vi "Value with no SI Prefix To Value with SI prefix.vi"(7 "Output Prefix":T1, 8 "error in":errorcluster, 10 "Unit In":T2, 11 "Scaled Value":dbl format="%#.6f") -> (0 "error out":errorcluster, 2 "Unit (with prefix)":T2, 3 "Value":dbl format="%#.6f")   [LabVIEW 2013, in "Mercury iXX.lvlib"]
doc: "This VI converts a numeric input in base units into a numeric with a user-selectable SI prefix."
uses:
  <instrlib>/Mercury iXX/Mercury iXX.lvlib
  <instrlib>/Mercury iXX/Public/Controls/Unit String.ctl
  <instrlib>/Mercury iXX/Public/Controls/SI Prefix.ctl
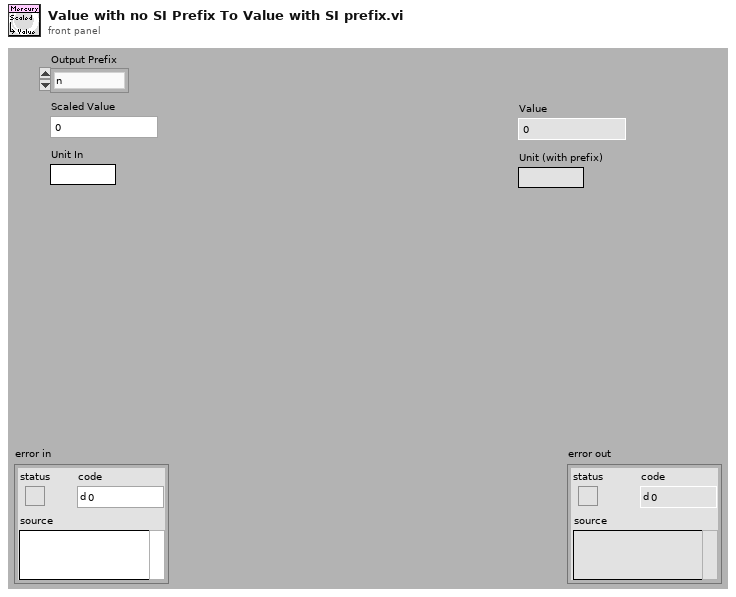
[diagram p1: front panel]
types:
  T1 = typedef "Mercury iXX.lvlib/SI Prefix.ctl" = enum16{"n", "µ", "m", "No Prefix", "k", "M", "G"}
  T2 = typedef "Mercury iXX.lvlib/Unit String.ctl" = string
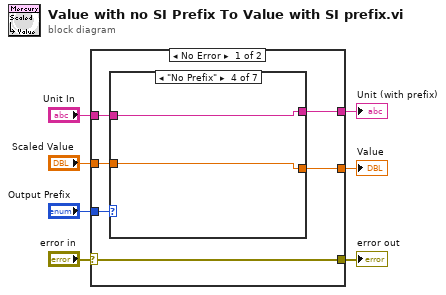
[diagram p0: block diagram]
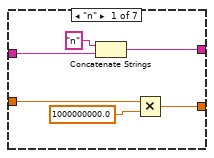
[diagram p2: hidden frame]
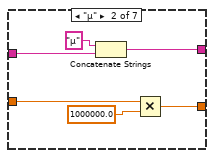
[diagram p3: hidden frame]
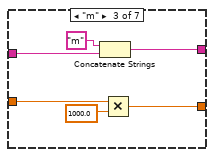
[diagram p4: hidden frame]
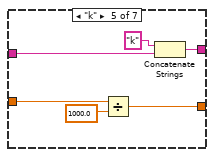
[diagram p5: hidden frame]
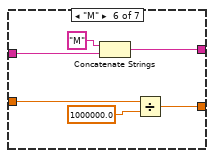
[diagram p6: hidden frame]
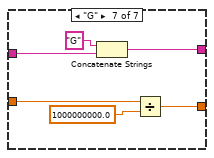
[diagram p7: hidden frame]
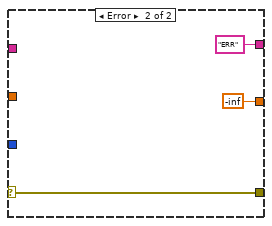
[diagram p8: hidden frame]
diagram:
  n1 = case shown="No Error" "error in" {
    selector: "error in" -> [w8 w54]
    tunnel: [w8 w54] -> w6
    tunnel: [w13 -inf] -> w5
    tunnel: [w9 "ERR" ("Unit-")] -> w4
    tunnel: "Scaled Value" -> [w12 _]
    tunnel: "Output Prefix" -> [w11 _]
    tunnel: "Unit In" -> [w10 _]
    frame No Error {
      n2 = case shown="\"No Prefix\"" w11 {
        tunnel: [w14 w24 w30 w32 w38 w44 w49] -> w13
        tunnel: w12 -> [w17 w23 w29 w32 w37 w43 w50]
        tunnel: w10 -> [w16 w20 w26 w33 w34 w40 w46]
        tunnel: [w15 w22 w28 w33 w36 w42 w48] -> w9
        frame "n" {
          n3 = Concatenate Strings("n" ("string"), w16) -> (w15:string)
          n4 = Multiply(x=w17, y=1000000000.0) -> (x*y=w14:dbl)
        }
        frame "µ" {
          n5 = Concatenate Strings("µ" ("string"), w20) -> (w22:string)
          n6 = Multiply(x=w23, y=1000000.0) -> (x*y=w24:dbl)
        }
        frame "m" {
          n7 = Concatenate Strings("m" ("string"), w26) -> (w28:string)
          n8 = Multiply(x=w29, y=1000.0) -> (x*y=w30:dbl)
        }
        frame "No Prefix" {
        }
        frame "k" {
          n9 = Divide(x=w37, y=1000.0) -> (x/y=w38:dbl)
          n10 = Concatenate Strings("k" ("string"), w34) -> (w36:string)
        }
        frame "M" {
          n11 = Concatenate Strings("M" ("string"), w40) -> (w42:string)
          n12 = Divide(x=w43, y=1000000.0) -> (x/y=w44:dbl)
        }
        frame "G" {
          n13 = Concatenate Strings("G" ("string"), w46) -> (w48:string)
          n14 = Divide(x=w50, y=1000000000.0) -> (x/y=w49:dbl)
        }
      }
    }
    frame Error {
    }
  }
  "error out" <- w6
  "Value" <- w5
  "Unit (with prefix)" <- w4
